vi "Write Key (Path).vi"(7 "section":string caption="Abschnitt", 8 "error in (no error)":errorcluster caption="Fehler (Eingang, kein Fehler)", 9 "value":path caption="Wert", 10 "key":string caption="Schlüssel", 11 "refnum":T1 caption="RefNum") -> (0 "error out":errorcluster caption="Fehler (Ausgang)", 3 "refnum out":T1 caption="RefNum (Ausgang)")   [LabVIEW 2009]
doc: "Schreibt einen Wert, der einem Schlüssel in einem angegebenen Abschnitt in der durch <B>Refnum</B> angegebenen Konfigurationsdatei zugeordnet ist. Mit diesem polymorphen VI können folgende Wertetypen in einen Schlüssel geschrieben werden: boolesche Werte, numerische Werte mit doppelter Genauigkeit, vorzeichenbehaftete Integer-Werte, Pfade, Strings und vorzeichenlose Integer-Werte. Durch den Datentypen, der am Eingang <B>Wert</B> anliegt, wird festgelegt, welche Funktion das polymorphe VI ausführen soll."
uses:
  <vilib>/Utility/config.llb/Config Data RefNum.ctl
  Config Data Modify Functions.ctl
  <vilib>/Utility/config.llb/NI_LVConfig.lvlib
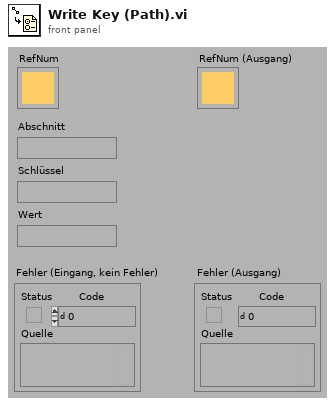
[diagram p1: front panel]
types:
  T1 = typedef "NI_LVConfig.lvlib/Config Data RefNum.ctl" = refnum<k1>
  T2 = typedef "Config Data Modify Functions.ctl" = enum16{"set file path", "put data", "add key", "remove section", "remove key"}
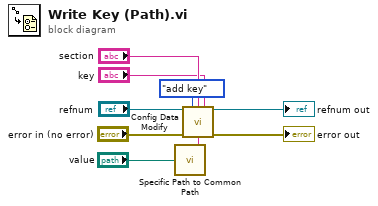
[diagram p0: block diagram]
diagram:
  n1 = call "Specific Path to Common Path.vi"("specific path"="value") -> ("common path"=w4:string)  [unwired: 4 in]
  n2 = call "Config Data Modify.vi"("config data"="refnum", "function"=Config_Data_Modify_Functions."add key", "section"="section", "key"="key", "error in (no error)"="error in (no error)", "value"=w4) -> ("config data out"=→"refnum out":T1, "error out"=→"error out":errorcluster)  [unwired: 6 in, 2 out]
